vi "从配置文件获取企业信息.vi"(10 "登录名":string) -> (0 "error out":errorcluster caption="错误输出", 2 "企业信息":T1)   [LabVIEW 2013, in "个人剂量仪-云服务器.lvclass"]
uses:
  <vilib>/Utility/config.llb/Read Key (String).vi
  <vilib>/Utility/config.llb/NI_LVConfig.lvlib
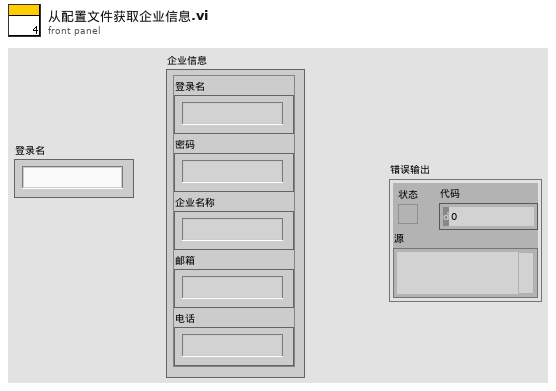
[diagram p1: front panel]
types:
  T1 = cluster{"登录名":string, "密码":string, "企业名称":string, "邮箱":string, "电话":string}
  T2 = typedef "NI_LVConfig.lvlib/Config Data RefNum.ctl" = refnum<k1>
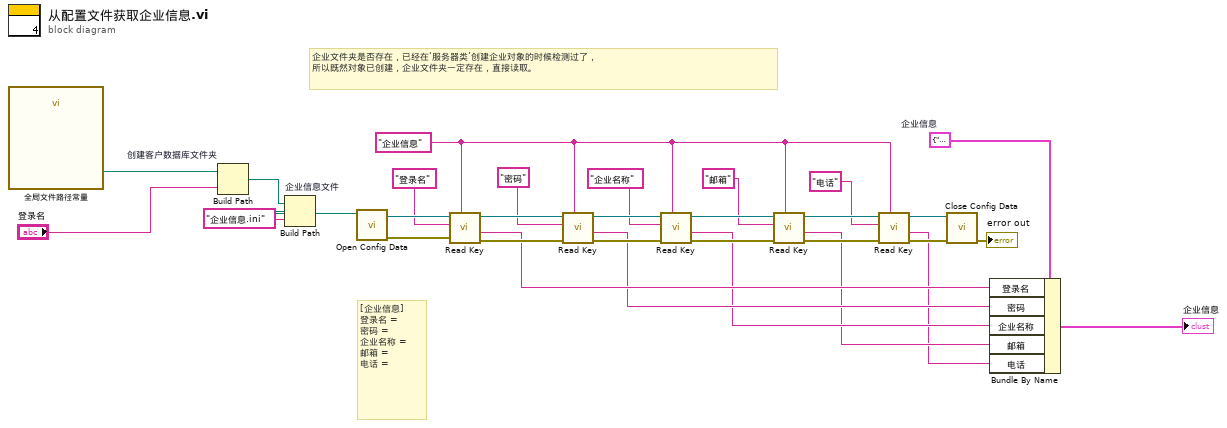
[diagram p0: block diagram]
diagram:
  w15 = T1 {"登录名"="", "密码"="", "企业名称"="", "邮箱"="", "电话"=""}  # 企业信息
  w21 = "企业信息" ("section")
  # "[企业信息]\n登录名 = \n密码 = \n企业名称 = \n邮箱 = \n电话 ="
  # "企业文件夹是否存在，已经在‘服务器类’创建企业对象的时候检测过了，\n所以既然对象已创建，企业文件夹一定存在，直接读取。"
  n1 = call "全局文件路径常量.vi"() -> ("用户数据库根目录"=w31:path)  [unwired: 9 in, 2 out]
  n2 = Build Path "创建客户数据库文件夹"(base path=w31, name or relative path="登录名") -> (appended path=w28:path)
  n3 = Build Path "企业信息文件"(base path=w28, name or relative path="企业信息.ini" ("名称或相对路径")) -> (appended path=w27:path)
  n4 = call <vilib>:"Open Config Data.vi"("configuration file path"=w27) -> ("error out"=w12:errorcluster, "refnum"=w26:T2)  [unwired: 8 in, 1 out]
  n5 = call-poly <vilib>:"Read Key.vi"("section"=w21, "error in (no error)"=w12, "key"="登录名" ("section"), "refnum"=w26) -> ("error out"=w13:errorcluster, "value"=w7:string, "refnum out"=w25:T2)  [unwired: 4 in, 1 out]
  n6 = call-poly <vilib>:"Read Key.vi"("section"=w21, "error in (no error)"=w13, "key"="密码" ("section"), "refnum"=w25) -> ("error out"=w11:errorcluster, "value"=w6:string, "refnum out"=w24:T2)  [unwired: 4 in, 1 out]
  n7 = call-poly <vilib>:"Read Key.vi"("section"=w21, "error in (no error)"=w11, "key"="企业名称" ("section"), "refnum"=w24) -> ("error out"=w10:errorcluster, "value"=w5:string, "refnum out"=w23:T2)  [unwired: 4 in, 1 out]
  n8 = call-poly <vilib>:"Read Key.vi"("section"=w21, "error in (no error)"=w10, "key"="邮箱" ("section"), "refnum"=w23) -> ("error out"=w9:errorcluster, "value"=w4:string, "refnum out"=w22:T2)  [unwired: 4 in, 1 out]
  n9 = call-poly <vilib>:"Read Key.vi"("section"=w21, "error in (no error)"=w9, "key"="电话" ("section"), "refnum"=w22) -> ("error out"=w8:errorcluster, "value"=w3:string, "refnum out"=w14:T2)  [unwired: 4 in, 1 out]
  n10 = call <vilib>:"Close Config Data.vi"("error in (no error)"=w8, "refnum"=w14) -> ("error out"=→"error out":errorcluster)  [unwired: 8 in, 1 out]
  n11 = Bundle By Name(cluster=w15, "登录名"=w7, "密码"=w6, "企业名称"=w5, "邮箱"=w4, "电话"=w3) -> (→"企业信息":T1)
